vi "STOP.vi"(8 "error in (no error)":errorcluster, 11 "Stop in":refnum<class "Avantes_bunch.lvclass">) -> (0 "error out":errorcluster, 3 "Stop out":refnum<class "Avantes_bunch.lvclass">)   [LabVIEW 2020, in "Avantes_bunch.lvclass"]
uses:
  Avantes_bunch.lvclass
  C:/Dev/TRANCON/Classes/GeneralFunctionality/GeneralFunctionality.lvclass
  Avantes_bunch.lvclass/Avantes_bunch.ctl
  GeneralFunctionality/GeneralFunctionality.lvclass/GeneralFunctionality.ctl
  Detector.lvclass
  GeneralFunctionality/GeneralFunctionality.lvclass
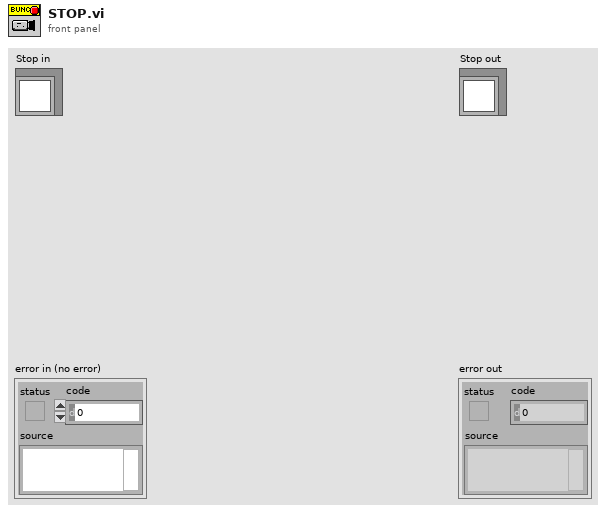
[diagram p1: front panel]
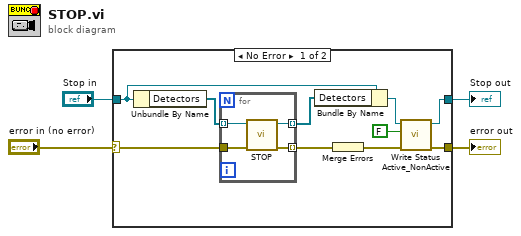
[diagram p0: block diagram]
diagram:
  n1 = case shown="No Error" "error in (no error)" {
    selector: "error in (no error)" -> [w13 w20]
    tunnel: [w6 w20] -> w3
    tunnel: [w5 w19] -> w2
    tunnel: "Stop in" -> [w12 w19]
    frame No Error {
      n2 = Unbundle By Name(w12) -> ("Detectors"=w14:refnum<class "Detector.lvclass">[])
      n3 = for {
        tunnel: w14 -> [w18] mode=indexing
        tunnel: w13 -> [w17]
        tunnel: [w16] -> w8 mode=indexing
        tunnel: [w15] -> w11 mode=indexing
        n4 = call-dynamic "STOP.vi"("error in (no error)"=w17, "Stop in"=w18) -> ("error out"=w16:errorcluster, "Stop out"=w15:refnum<class "Detector.lvclass">)  [unwired: 8 in]
      }
      n5 = Bundle By Name(cluster=w12, "Detectors"=w11) -> (w10:refnum<class "Avantes_bunch.lvclass">)
      n6 = Merge Errors(w8) -> (w7:errorcluster)
      n7 = call "Write Status Active_NonActive.vi"("error in (no error)"=w7, "Status Active/NonActive"=FALSE, "GeneralFunctionality in"=w10) -> ("error out"=w6:errorcluster, "GeneralFunctionality out"=w5:refnum<class "Avantes_bunch.lvclass">)  [unwired: 7 in]
    }
    frame Error {
    }
  }
  "error out" <- w3
  "Stop out" <- w2
